vi "Test Customer Pick Up Last Order Item Stops.vi"(8 "error in (no error)":errorcluster, 11 "Customer Test in":refnum<class "Customer Test.lvclass">) -> (0 "error out":errorcluster, 3 "Customer Test out":refnum<class "Customer Test.lvclass">)   [LabVIEW 2020, in "Customer Test.lvclass"]
uses:
  Customer Test.lvclass
  C:/Program Files (x86)/National Instruments/LabVIEW 2020/vi.lib/Asteme/LUnit/Test Case.lvclass
  Processes/People/Customers/Customer/Customer.lvclass
  C:/Program Files (x86)/National Instruments/LabVIEW 2020/vi.lib/Asteme/Triarc Framework/Process/Process.lvclass
  Support/Beverages/Beverage/Beverage.lvclass
  Support/Beverages/TypeDefs/Drink Type.ctl
  Support/Beverages/TypeDefs/Options.ctl
  <vilib>/Asteme/Triarc Framework/Process/Public/Lifecycle/Lifecycle State.ctl
  Test Doubles/Stub Job Handler/Stub Job Handler.lvclass
  C:/Users/anton/Documents/GitHub/Triarc-Examples/Coffee Shop/Process Job/Job Handler.lvclass
  <vilib>/Asteme/LUnit/Test Case.lvclass/Test Case.ctl
  <vilib>/Asteme/LUnit/LUnit Assertion Result.lvclass/LUnit Assertion Result.ctl
  <vilib>/Asteme/LUnit/Palette/Pass If.vi
  <vilib>/Asteme/LUnit/Set Assertion Type.vi
  <vilib>/Asteme/LUnit/Palette/Fail.vi
  <vilib>/Asteme/LUnit/Palette/Pass.vi
  <vilib>/Asteme/LUnit/LUnit Write Assertion Type.vi
  <vilib>/Asteme/LUnit/Add test result.vi
  <vilib>/Asteme/LUnit/LUnit Write Passed.vi
  <vilib>/Asteme/LUnit/LUnit Get Test Case.vi
  <vilib>/Asteme/LUnit/Assertion Result/LUnit Get Test Name.vi
  <vilib>/Asteme/LUnit/LUnit Write Message.vi
  <vilib>/Asteme/LUnit/LUnit Write Description.vi
  <vilib>/Asteme/LUnit/Read Test Case Name.vi
  <vilib>/Asteme/LUnit/LUnit Assertion Result.lvclass
  <vilib>/Asteme/Triarc Framework/Process/Process.lvclass
  <vilib>/Asteme/LUnit/Test Case.lvclass
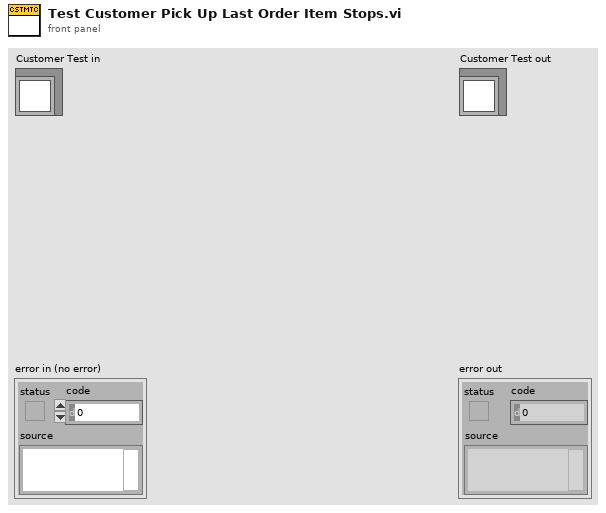
[diagram p1: front panel]
types:
  T1 = typedef "TF.lvlib/Process.lvclass/Lifecycle State.ctl" = enum16{"Uninitialized", "Initialized", "Started", "Running", "Stopped", "Finished"}
  T2 = typedef "Beverage.lvclass/Drink Type.ctl" = enum16{"Dark Roast", "Decaf", "Espresso", "House Blend"}
  T3 = typedef "Beverage.lvclass/Options.ctl" = enum16{"<None>", "Milk", "Mocha", "Soy", "Whip"}
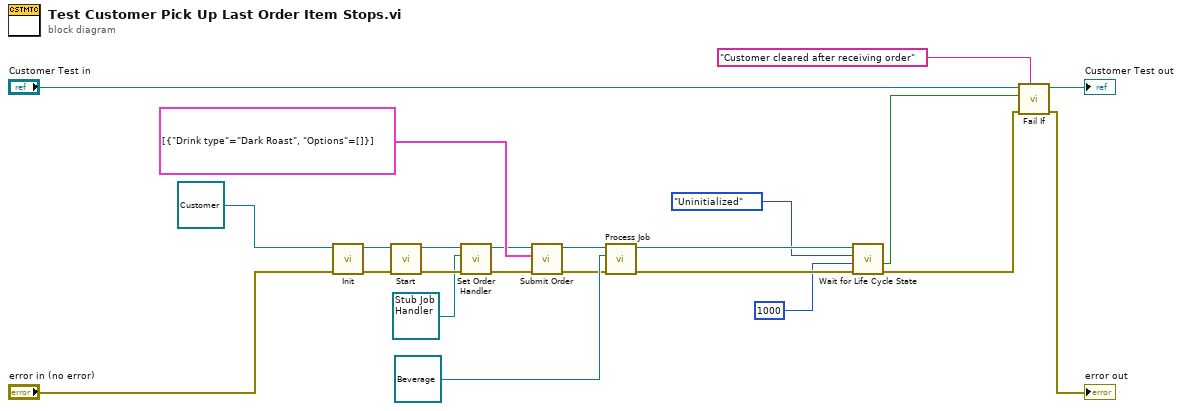
[diagram p0: block diagram]
diagram:
  n1 = call-dynamic "Init.vi"("error in (no error)"="error in (no error)", "View In"=refnum<class "Customer.lvclass"> refnum ("Customer.lvclass")) -> ("error out"=w21:errorcluster, "View Out"=w22:refnum<class "Customer.lvclass">)  [unwired: 8 in]
  n2 = call <vilib>:"Start.vi"("error in (no error)"=w21, "Process In"=w22) -> ("error out"=w19:errorcluster, "Process Out"=w3:refnum<class "Customer.lvclass">)  [unwired: 8 in]
  n3 = call "Set Order Handler.vi"("error in (no error)"=w19, "Order Handler"=refnum<class "Stub Job Handler.lvclass"> refnum ("Stub Job Handler.lvclass"), "Customer In"=w3) -> ("error out"=w4:errorcluster, "Customer Out"=w2:refnum<class "Customer.lvclass">)  [unwired: 7 in]
  n4 = call "Submit Order.vi"("error in (no error)"=w4, "Order Content"=cluster{"Drink type":T2, "Options":T3[]}[] [{"Drink type"=enum."Dark Roast", "Options"=[]}], "Customer In"=w2) -> ("error out"=w10:errorcluster, "Customer Out"=w9:refnum<class "Customer.lvclass">)  [unwired: 7 in]
  n5 = call-dynamic "Process Job.vi"("error in (no error)"=w10, "Job"=refnum<class "Beverage.lvclass"> refnum ("Beverage.lvclass"), "Process Job In"=w9) -> ("error out"=w18:errorcluster, "Process Job Out"=w11:refnum<class "Customer.lvclass">)  [unwired: 7 in]
  n6 = call <vilib>:"Wait for Life Cycle State.vi"("error in (no error)"=w18, "timeout in ms (-1)"=1000, "Lifecycle State"=Lifecycle_State."Uninitialized", "Process In"=w11) -> ("error out"=w12:errorcluster, "timed out?"=w5:bool)  [unwired: 5 in, 1 out]
  n7 = call <vilib>:"Fail If.vi"("Description"="Customer cleared after receiving order", "error in (no error)"=w12, "Fail?"=w5, "Test Case In"="Customer Test in") -> ("error out"=→"error out":errorcluster, "Test Case Out"=→"Customer Test out":refnum<class "Customer Test.lvclass">)  [unwired: 6 in]
